vi "UUT - WLAN - WLM - UTIL - subVIs - MACStringToU64.vi"(0 "Address String":string, 11 "error in":errorcluster) -> (4 "Address U64":u64 format="%x", 15 "error out":errorcluster)   [LabVIEW 2011]
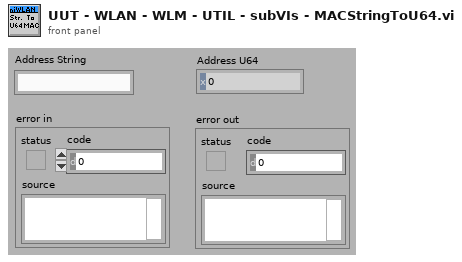
[diagram p1: front panel]
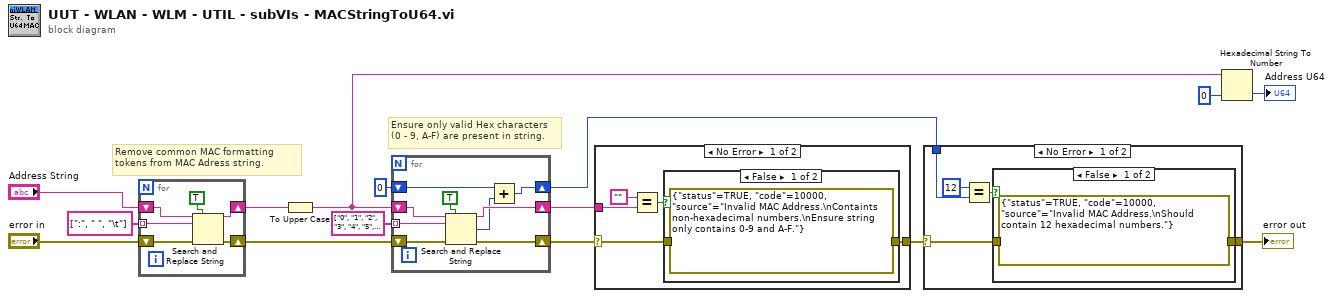
[diagram p0: block diagram]
diagram:
  # "Remove common MAC formatting\ntokens from MAC Adress string."
  # "Ensure only valid Hex characters\n(0 - 9, A-F) are present in string."
  n1 = for {
    tunnel: string[] [":", " ", "\t"] -> [w19] mode=indexing
    shift-right: [w20] -> w6
    shift-left: "Address String" -> [w21]
    shift-right: [w17] -> w7
    shift-left: "error in" -> [w18]
    n2 = Search and Replace String(replace all?=TRUE ("replace all? (F)"), input string=w21, search string=w19, error in=w18) -> (result string=w20:string, error out=w17:errorcluster)  [unwired: 6 out]
  }
  n3 = To Upper Case(1:w6) -> (0:w10:string)
  n4 = for {
    tunnel: string[] ["0", "1", "2", "3", "4", "5", "6", "7", "8", "9", "A", "B", "C", "D", "E", "F"] -> [w28] mode=indexing
    shift-right: [w29] -> w12
    shift-left: w10 -> [w30]
    shift-right: [w26] -> w5
    shift-left: w7 -> [w27]
    shift-right: [w22] -> w3
    shift-left: 0 ("number of replacements") -> [w24]
    n5 = Search and Replace String(replace all?=TRUE ("replace all? (F)"), input string=w30, search string=w28, error in=w27) -> (result string=w29:string, number of replacements=w23:i32, error out=w26:errorcluster)  [unwired: 5 out]
    n6 = Add(x=w24, y=w23) -> (x+y=w22:i32)
  }
  n7 = case shown="No Error" w5 {
    selector: w5 -> [w32 w38]
    tunnel: w12 -> [w35 _]
    tunnel: [w31 w38] -> w4
    frame No Error {
      n8 = Equal?(x="", y=w35) -> (x = y?=w33:bool)
      n9 = case shown="False" w33 {
        tunnel: w32 -> [_ w37]
        tunnel: [errorcluster {"status"=TRUE, "code"=10000, "source"="Invalid MAC Address.\nContaints non-hexadecimal numbers.\nEnsure string only contains 0-9 and A-F."} ("error IO") w37] -> w31
        frame False {
        }
        frame True {
        }
      }
    }
    frame Error {
    }
  }
  n10 = case shown="No Error" w4 {
    selector: w4 -> [w41 w46]
    tunnel: w3 -> [w42 _]
    tunnel: [w39 w46] -> w2
    frame No Error {
      n11 = Equal?(x=12, y=w42) -> (x = y?=w40:bool)
      n12 = case shown="False" w40 {
        tunnel: w41 -> [_ w45]
        tunnel: [errorcluster {"status"=TRUE, "code"=10000, "source"="Invalid MAC Address.\nShould contain 12 hexadecimal numbers."} ("error IO") w45] -> w39
        frame False {
        }
        frame True {
        }
      }
    }
    frame Error {
    }
  }
  "error out" <- w2
  n13 = Hexadecimal String To Number(string=w10, default (0uL)=u64 0 ("default (0 U32)")) -> (number=→"Address U64":u64)  [unwired: 2 out]
